vi "GSCS_PDA_FormStatusString.vi"(1 "System Info":T1) -> (0 "String":string)   [LabVIEW 2015]
uses:
  SystemInfoCluster.ctl
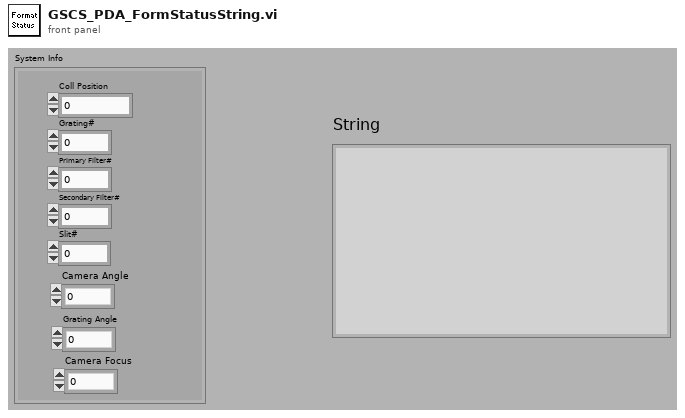
[diagram p1: front panel]
types:
  T1 = typedef "SystemInfoCluster.ctl" = cluster{"Coll Position":i32, "Grating#":i32, "Primary Filter#":i32, "Secondary Filter#":i32, "Slit#":i32, "Camera Angle":dbl, "Grating Angle":dbl, "Camera Focus":i32}
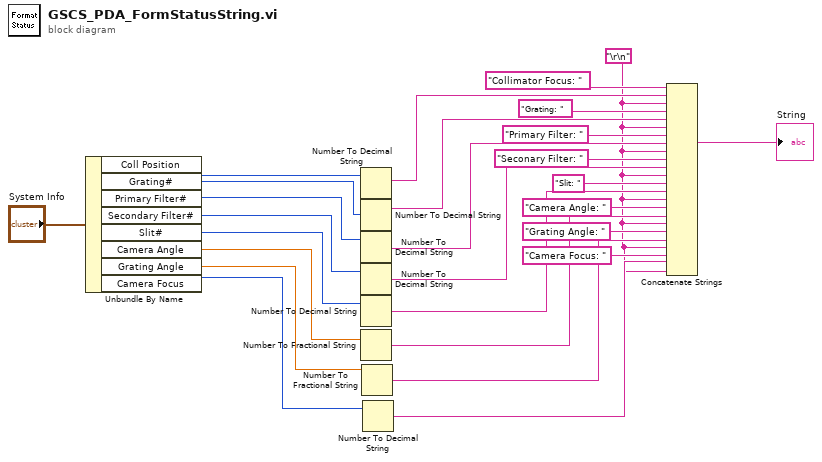
[diagram p0: block diagram]
diagram:
  w1 = "\r\n"
  n1 = Unbundle By Name("System Info") -> ("Coll Position"=w26:i32, "Grating#"=w25:i32, "Primary Filter#"=w24:i32, "Secondary Filter#"=w23:i32, "Slit#"=w22:i32, "Camera Angle"=w10:dbl, "Grating Angle"=w9:dbl, "Camera Focus"=w8:i32)
  n2 = Number To Decimal String(number=w26) -> (decimal integer string=w21:string)  [unwired: 1 in]
  n3 = Number To Decimal String(number=w25) -> (decimal integer string=w17:string)  [unwired: 1 in]
  n4 = Number To Decimal String(number=w24) -> (decimal integer string=w15:string)  [unwired: 1 in]
  n5 = Number To Decimal String(number=w23) -> (decimal integer string=w13:string)  [unwired: 1 in]
  n6 = Number To Decimal String(number=w22) -> (decimal integer string=w11:string)  [unwired: 1 in]
  n7 = Number To Fractional String(number=w10) -> (F-format string=w6:string)  [unwired: 3 in]
  n8 = Number To Fractional String(number=w9) -> (F-format string=w4:string)  [unwired: 3 in]
  n9 = Number To Decimal String(number=w8) -> (decimal integer string=w2:string)  [unwired: 1 in]
  n10 = Concatenate Strings("Collimator Focus: ", w21, w1, "Grating: ", w17, w1, "Primary Filter: ", w15, w1, "Seconary Filter: ", w13, w1, "Slit: ", w11, w1, "Camera Angle: " ("string"), w6, w1, "Grating Angle: " ("string"), w4, w1, "Camera Focus: " ("string"), w2, w1) -> (→"String":string)
